vi "Untitled 3.vi"() -> ()   [LabVIEW 2018]
uses:
  <instrlib>/RIGOL DS1000 Series/RIGOL DS1000 Series.lvlib
panel:
  out "Measured Value":dbl
  in  "VISA Oscilloscope":refnum<visa-resource-name>
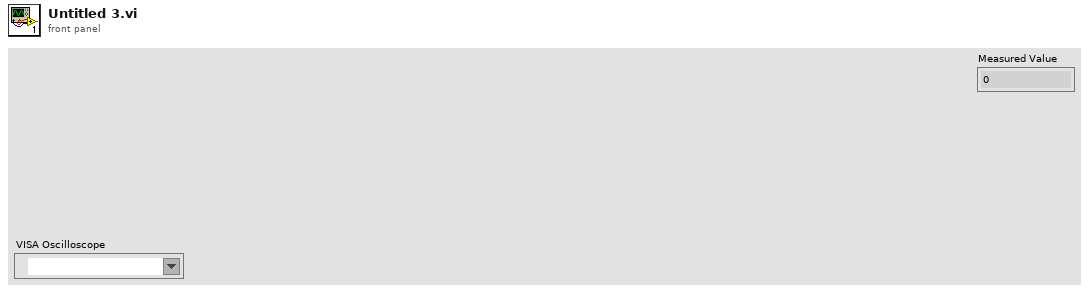
[diagram p1: front panel]
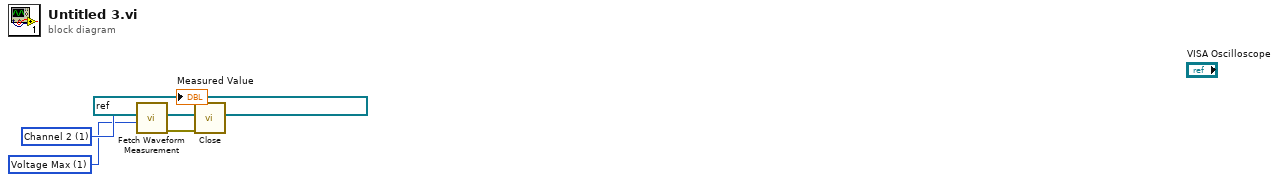
[diagram p0: block diagram]
diagram:
  w4 = u16 1 items=["Voltage Vpp", "Voltage Max", "Voltage Min", "Amplitude", "Voltage TOP", "Voltage Base", "Voltage Average", "Voltage RMS", "Overshoot", "Preshoot", "Frequency", "Rise Time", "Fall Time", "Period", "Positive Width", "Negative Width", "Positive Duty", "Negative Duty"] ("Measurement Function (0: Voltage Vpp)")
  w5 = u16 1 items=["Channel 1", "Channel 2", "Channel 3", "Channel 4"] ("Channel (0: Channel 1)")
  n1 = call <instrlib>:"Fetch Waveform Measurement.vi"("Measurement Function (0: Voltage Vpp)"=w4, "Source (0: Channel 1)"=w5, "VISA resource name"=refnum<visa-resource-name> "USB0::0x1AB1::0x0488::DS1BA202100064::INSTR") -> ("error out"=w6:errorcluster, "Measured Value"=→"Measured Value":dbl, "VISA resource name out"=w3:refnum<visa-resource-name>)  [unwired: 6 in]
  n2 = call <instrlib>:"Close.vi"("error in (no error)"=w6, "VISA resource name"=w3) -> ()  [unwired: 9 in, 1 out]
